vi "getCamPrefs.vi"(8 "Error In":errorcluster, 11 "INIfilePath":path) -> (0 "Error Out":errorcluster, 2 "Array":T1[](array[typedef]))   [LabVIEW 2021]
uses:
  camCluster.ctl
  <vilib>/Utility/config.llb/Read Key (String).vi
  <vilib>/Utility/config.llb/NI_LVConfig.lvlib
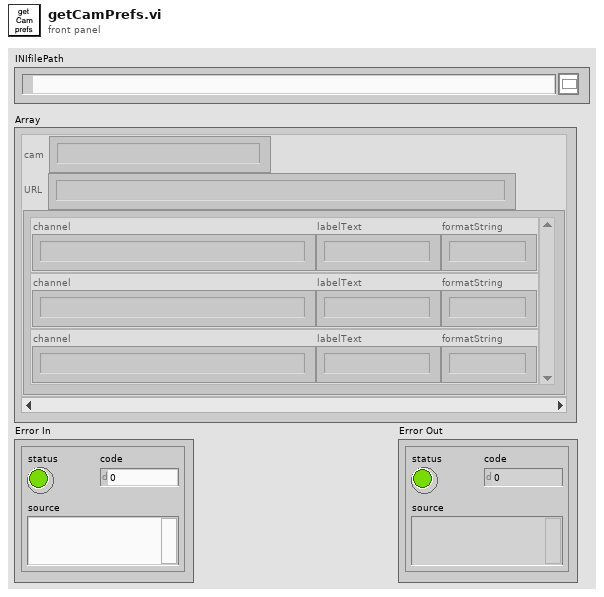
[diagram p1: front panel]
types:
  T1 = typedef "camCluster.ctl" = cluster{"cam":string, "URL":string, "ADAMspecs":cluster{"channel":string, "labelText":string, "formatString":string}[]}
  T2 = typedef "NI_LVConfig.lvlib/Config Data RefNum.ctl" = refnum<k1>
  T3 = cluster{"string array[0]":string, "string array[1]":string, "string array[2]":string}
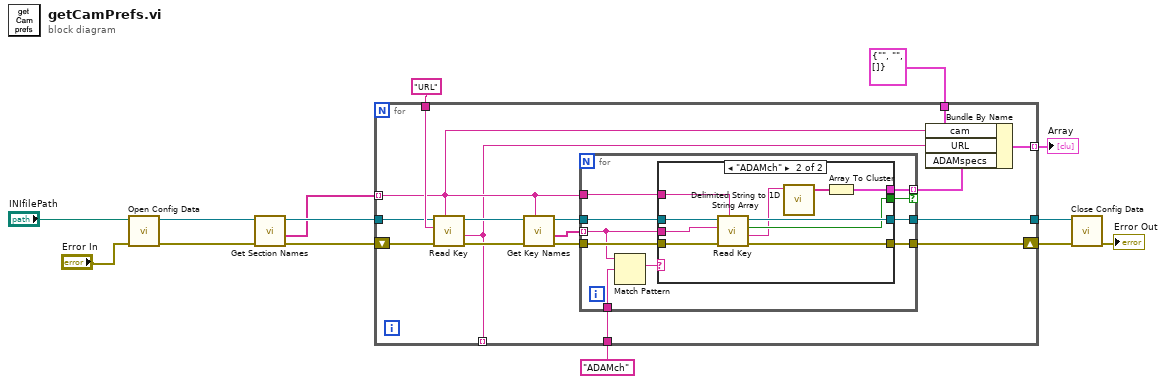
[diagram p0: block diagram]
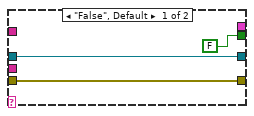
[diagram p2: hidden frame]
diagram:
  n1 = call <vilib>:"Open Config Data.vi"("error in (no error)"="Error In", "configuration file path"="INIfilePath") -> ("error out"=w12:errorcluster, "refnum"=w14:T2)  [unwired: 7 in, 1 out]
  n2 = call <vilib>:"Get Section Names.vi"("error in (no error)"=w12, "refnum"=w14) -> ("error out"=w8:errorcluster, "section names"=w5:string[], "refnum out"=w10:T2)  [unwired: 7 in]
  n3 = for {
    tunnel: w5 -> [w18] mode=indexing
    tunnel: w10 -> [w26]
    tunnel: [w28] -> w9
    tunnel: [w17] -> _ mode=indexing
    shift-right: [w27] -> w7
    shift-left: w8 -> [w30]
    tunnel: "URL" ("key") -> [w29]
    tunnel: "ADAMch" ("key") -> [w20]
    tunnel: T1 {"cam"="", "URL"="", "ADAMspecs"=[]} ("camCluster") -> [w19]
    tunnel: [w16] -> w1 mode=indexing
    n4 = call-poly <vilib>:"Read Key.vi"("section"=w18, "error in (no error)"=w30, "key"=w29, "refnum"=w26) -> ("error out"=w24:errorcluster, "value"=w17:string, "refnum out"=w25:T2)  [unwired: 4 in, 1 out]
    n5 = call <vilib>:"Get Key Names.vi"("section"=w18, "error in (no error)"=w24, "refnum"=w25) -> ("error out"=w22:errorcluster, "key names"=w21:string[], "refnum out"=w23:T2)  [unwired: 5 in, 1 out]
    n6 = for {
      tunnel: w18 -> [w36]
      tunnel: w21 -> [w33] mode=indexing
      tunnel: w23 -> [w38]
      tunnel: [w40] -> w28
      tunnel: w22 -> [w37]
      tunnel: [w39] -> w27
      tunnel: w20 -> [w34]
      tunnel: [w32] -> w15 mode=indexing if=w31
      n7 = Match Pattern(string=w33, regular expression=w34) -> (match substring=w35:string)  [unwired: 1 in, 3 out]
      n8 = case shown="\"ADAMch\"" w35 {
        tunnel: [w43 w53] -> w40
        tunnel: [w42 w52] -> w39
        tunnel: w38 -> [w43 w51]
        tunnel: w37 -> [w42 w50]
        tunnel: w36 -> [_ w49]
        tunnel: w33 -> [_ w48]
        tunnel: [_ w44] -> w32
        tunnel: [FALSE w47] -> w31
        frame "False", Default {
        }
        frame "ADAMch" {
          n9 = call-poly <vilib>:"Read Key.vi"("section"=w49, "error in (no error)"=w50, "key"=w48, "refnum"=w51) -> ("error out"=w52:errorcluster, "value"=w46:string, "found?"=w47:bool, "refnum out"=w53:T2)  [unwired: 4 in]
          n10 = call <vilib>:"Delimited String to 1D String Array.vi"("delimited string"=w46) -> ("string array"=w45:string[])  [unwired: 10 in]
          n11 = Array To Cluster(array=w45) -> (cluster=w44:T3)
        }
      }
    }
    n12 = Bundle By Name(cluster=w19, "cam"=w18, "URL"=w17, "ADAMspecs"=w15) -> (w16:T1)
  }
  "Array" <- w1
  n13 = call <vilib>:"Close Config Data.vi"("error in (no error)"=w7, "refnum"=w9) -> ("error out"=→"Error Out":errorcluster)  [unwired: 8 in, 1 out]
